vi "zad6.vi"() -> ()   [LabVIEW 2018]
panel:
  in  "?":bool
  out "Time Signal":waveform(dbl)[](graph)
  in  "file path":path
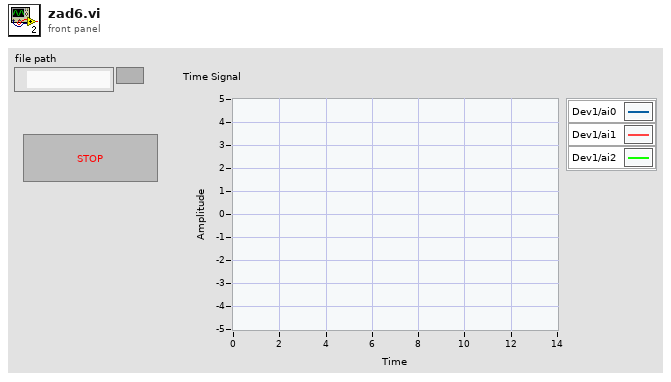
[diagram p1: front panel]
types:
  T1 = enum16{"open", "open or create", "create or replace", "create", "open (read-only)"}
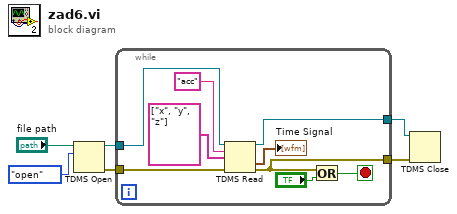
[diagram p0: block diagram]
diagram:
  n1 = TDMS Open(10:T1."open" ("operation (0:open)"), 11:"file path") -> (0:w2:errorcluster, 3:w4:refnum<k34>)  [unwired: 5 in]
  n2 = while {
    tunnel: w4 -> [w15]
    tunnel: [w14] -> w3
    tunnel: w2 -> [w13]
    tunnel: [w8] -> w1
    stop <- w9 stop-if-true
    n3 = TDMS Read(0:w15, 5:"acc" ("group name in"), 7:string[] ["x", "y", "z"] ("channel name(s) in"), 11:w13) -> (4:w14:refnum<k34>, 10:→"Time Signal":waveform(dbl)[], 15:w8:errorcluster)  [unwired: 4 in, 3 out]
    n4 = Or(x=w8, y="?") -> (x .or. y?=w9:bool)
  }
  n5 = TDMS Close(8:w1, 11:w3) -> ()  [unwired: 2 out]
